vi "Local Client.vi"(6 "timeout (ms) [500]":i32=500, 7 "type":variant, 8 "error in (no error)":errorcluster, 9 "params":variant, 10 "Command in":string, 11 "Instrument in":refnum<class "Instrument.lvclass">) -> (0 "error out":errorcluster, 1 "Data out":variant, 2 "Command out":string, 3 "Instrument out":refnum<class "Instrument.lvclass">)   [LabVIEW 2019, in "Instrument.lvclass"]
uses:
  Instrument.lvclass
  Local Client.vim/f183581a-e76b-4100-b83d-1a5040ff8dc4.vi/1015ab55-9266-47a6-9f37-a1dc735a0ade.vi
  Local Client.vim/f183581a-e76b-4100-b83d-1a5040ff8dc4.vi/15ff53cc-9836-4019-90a2-230f5451f966.vi
  <vilib>/Utility/Data Type/Get Type Information.vi
  <vilib>/JDP Science/JSONtext/JSON text to Variant.vi
  <vilib>/JDP Science/JSONtext/LVClass Serializer/JSONtext LVClass Serializer.lvclass
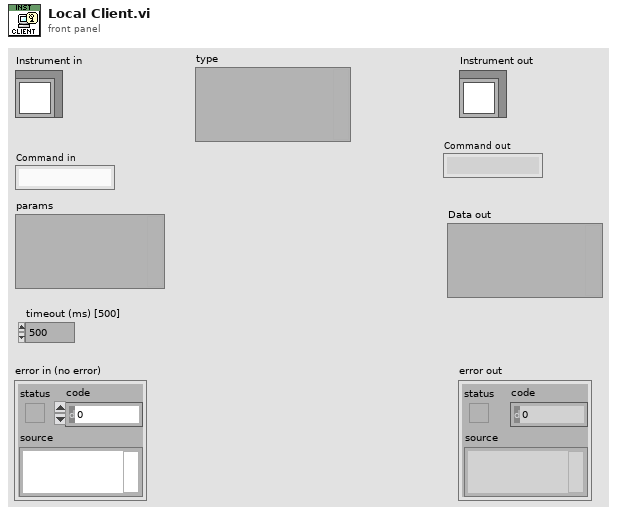
[diagram p1: front panel]
types:
  T1 = typedef "Instrument.lvclass/PublicEvents--Cluster.ctl" = cluster{"MessageFromProcess":refnum<user-event>}
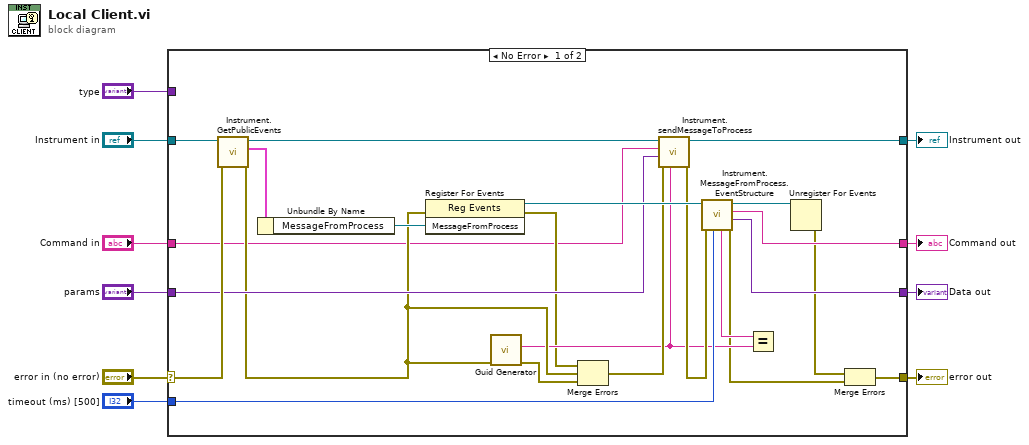
[diagram p0: block diagram]
diagram:
  n1 = case shown="No Error" "error in (no error)" {
    selector: "error in (no error)" -> [w27 w37]
    tunnel: [w11 w37] -> w9
    tunnel: [w33 w36] -> w7
    tunnel: "Instrument in" -> [w29 w36]
    tunnel: "Command in" -> [w16 w35]
    tunnel: "params" -> [w20 w34]
    tunnel: "timeout (ms) [500]" -> [w22 _]
    tunnel: [w15 w35] -> w3
    tunnel: [w14 w34] -> w2
    tunnel: "type" -> [_ _]
    frame No Error {
      n2 = call "Instrument.GetPublicEvents.vi"("error in (no error)"=w27, "Instrument"=w29) -> ("error out"=w19:errorcluster, "Instrument Public Events"=w32:T1, "Instrument out"=w28:refnum<class "Instrument.lvclass">)  [unwired: 7 in]
      n3 = Unbundle By Name(w32) -> ("MessageFromProcess"=w31:refnum<user-event>)
      n4 = register-events(error in=w19, w31) -> (reference out=w30:refnum<event-registration>, error out=w17:errorcluster)  [unwired: 1 in]
      n5 = call <vilib>:"Guid Generator.vi"("error in (no error)"=w19) -> ("error out"=w21:errorcluster, "GUID"=w18:string)  [unwired: 9 in]
      n6 = Merge Errors(w17, w19, w21) -> (w25:errorcluster)
      n7 = call "Instrument.sendMessageToProcess.vi"("ID"=w18, "error in (no error)"=w25, "Data"=w20, "Command"=w16, "Instrument"=w28) -> ("error out"=w24:errorcluster, "Instrument out"=w33:refnum<class "Instrument.lvclass">)  [unwired: 5 in]
      n8 = call "Instrument.MessageFromProcess.EventStructure.vi"("timeout (ms) [500]"=w22, "error in (no error)"=w24, "Event Registration Refnum in"=w30) -> ("error out"=w13:errorcluster, "Data"=w14:variant, "Command"=w15:string, "Event Registration Refnum out"=w26:refnum<event-registration>, "ID"=w23:string)  [unwired: 4 in]
      n9 = Equal?(x=w23, y=w18) -> ()  [unwired: 1 out]
      n10 = Unregister For Events(event registration refnum=w26) -> (error out=w12:errorcluster)  [unwired: 1 in]
      n11 = Merge Errors(w12, w13) -> (w11:errorcluster)
    }
    frame Error {
      # "leave unwired,\notherwise malleable VI\nwon't adapt properly"
    }
  }
  "error out" <- w9
  "Instrument out" <- w7
  "Command out" <- w3
  "Data out" <- w2
